vi "Subscribe.vi"(0 "STOMP in":refnum<class "STOMP.lvclass">, 1 "Destination":string, 2 "ack":T2, 3 "headers":T1[](array[typedef]), 5 "error in (no error)":errorcluster, 6 "Receipt?":bool) -> (14 "STOMP out":refnum<class "STOMP.lvclass">, 19 "error out":errorcluster)   [LabVIEW 2017, in "LabVIEW STOMP.lvlib" / "STOMP.lvclass"]
uses:
  STOMP.lvclass
  Typedefs/Type_AckHeader.ctl
  Typedefs/Type_FrameHeader.ctl
  Typedefs/Type_ClientFrameType.ctl
  Typedefs/Type_ClientFrame.ctl
  STOMP.lvclass/STOMP.ctl
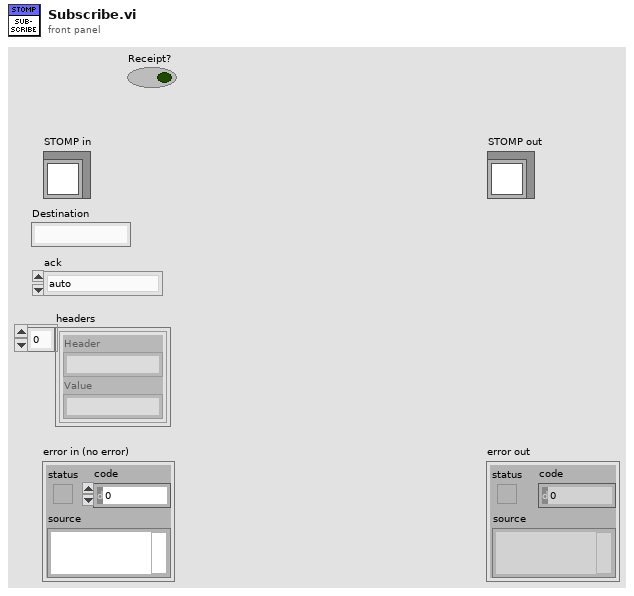
[diagram p1: front panel]
types:
  T1 = typedef "LabVIEW STOMP.lvlib/STOMP.lvclass/Type_FrameHeader.ctl" = cluster{"Header":string, "Value":string}
  T2 = typedef "Type_AckHeader.ctl" = enum16{"auto", "client", "client-individual"}
  T3 = typedef "LabVIEW STOMP.lvlib/STOMP.lvclass/Type_ClientFrame.ctl" = cluster{"Type":T4, "Headers":T1[], "Body":string}
  T4 = typedef "LabVIEW STOMP.lvlib/STOMP.lvclass/Type_ClientFrameType.ctl" = enum16{"Undefined", "SEND", "SUBSCRIBE", "UNSUBSCRIBE", "BEGIN", "COMMIT", "ABORT", "ACK", "NACK", "DISCONNECT"}
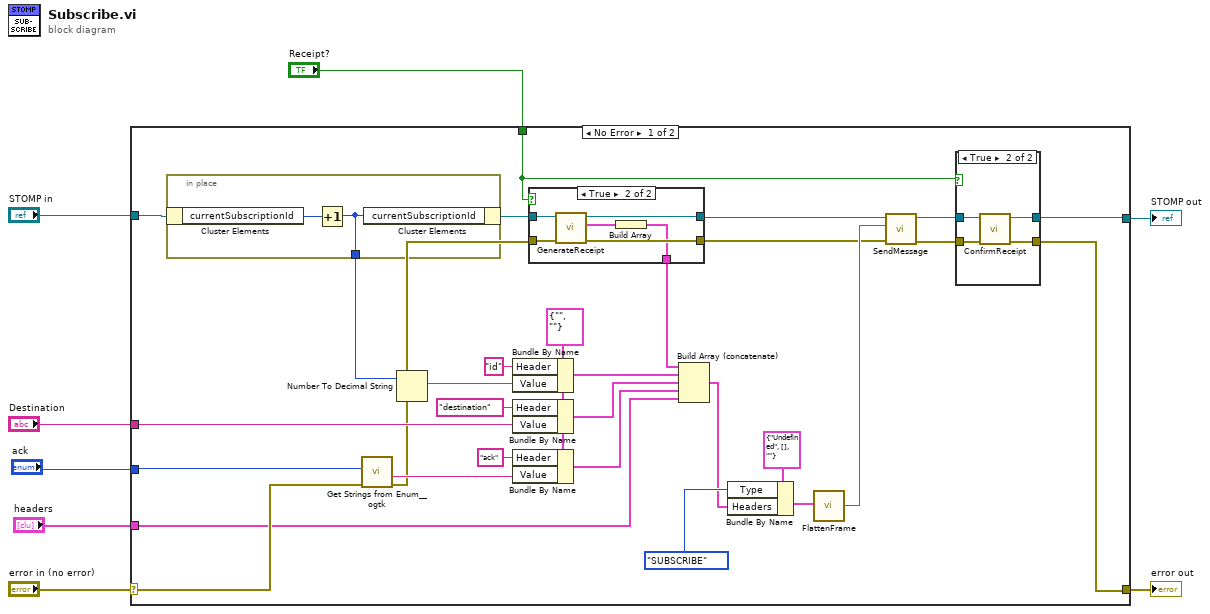
[diagram p0: block diagram]
diagram:
  n1 = case shown="No Error" "error in (no error)" {
    selector: "error in (no error)" -> [w24 w56]
    tunnel: [w16 w56] -> w7
    tunnel: [w17 w55] -> w5
    tunnel: "STOMP in" -> [w21 w55]
    tunnel: "Destination" -> [w33 _]
    tunnel: "ack" -> [w25 _]
    tunnel: "Receipt?" -> [w10 _]
    tunnel: "headers" -> [w9 _]
    frame No Error {
      w27 = T1 {"Header"="", "Value"=""}
      n2 = in-place {
        in-place-border: [w47] -> w31
        n3 = in-place-cluster #1(w21) -> ("currentSubscriptionId"=w48:u64)
        n4 = Increment(x=w48) -> (x+1=w47:u64)
        n5 = in-place-cluster #1("currentSubscriptionId"=w47) -> (w15:refnum<class "STOMP.lvclass">)
      }
      n6 = call <userlib>:"Get Strings from Enum__ogtk.vi"("error in (no error)"=w24, "Enum"=w25) -> ("error out"=w14:errorcluster, "String Value"=w23:string)  [unwired: 6 in, 2 out]
      n7 = Number To Decimal String(number=w31) -> (decimal integer string=w30:string)  [unwired: 1 in]
      n8 = Bundle By Name(cluster=w27, "Header"="id", "Value"=w30) -> (w29:T1)
      n9 = Bundle By Name(cluster=w27, "Header"="destination", "Value"=w33) -> (w28:T1)
      n10 = Bundle By Name(cluster=w27, "Header"="ack", "Value"=w23) -> (w22:T1)
      n11 = case shown="True" w10 {
        tunnel: w15 -> [w40 w46]
        tunnel: w14 -> [w39 w45]
        tunnel: [w40 w44] -> w11
        tunnel: [w39 w43] -> w12
        tunnel: [_ w41] -> w13
        frame False {
        }
        frame True {
          n12 = call-dynamic "GenerateReceipt.vi"("error in (no error)"=w45, "STOMP in"=w46) -> ("error out"=w43:errorcluster, "Receipt Header"=w42:T1, "STOMP out"=w44:refnum<class "STOMP.lvclass">)  [unwired: 7 in]
          n13 = Build Array(w42) -> (w41:T1[])
        }
      }
      n14 = Build Array (concatenate)(w13, w29, w28, w22, w9) -> (w35:T1[])
      n15 = Bundle By Name(cluster=T3 {"Type"=enum."Undefined", "Headers"=[], "Body"=""} ("Type_ClientFrame"), "Type"=Type_ClientFrameType."SUBSCRIBE", "Headers"=w35) -> (w34:T3)
      n16 = call "FlattenFrame.vi"("Client Frame"=w34) -> ("flattened frame"=w20:string)  [unwired: 18 in]
      n17 = call-dynamic "SendMessage.vi"("error in (no error)"=w12, "data in"=w20, "STOMP in"=w11) -> ("error out"=w18:errorcluster, "STOMP out"=w19:refnum<class "STOMP.lvclass">)  [unwired: 7 in]
      n18 = case shown="True" w10 {
        tunnel: w19 -> [w49 w54]
        tunnel: w18 -> [w50 w53]
        tunnel: [w50 w52] -> w16
        tunnel: [w49 w51] -> w17
        frame False {
        }
        frame True {
          n19 = call-dynamic "ConfirmReceipt.vi"("error in (no error)"=w53, "STOMP in"=w54) -> ("error out"=w52:errorcluster, "STOMP out"=w51:refnum<class "STOMP.lvclass">)  [unwired: 8 in]
        }
      }
    }
    frame Error {
    }
  }
  "error out" <- w7
  "STOMP out" <- w5
